vi "Get Joystick Output.vi"(0 "JoystickDevRef":T1={"Device"=enum."USB 1"}, 11 "error in (no error)":errorcluster) -> (3 "XBox?":bool, 4 "JoystickDevRef":T1, 6 "Axes":dbl[](array[numeric]), 8 "Buttons":bool[](array[boolean]), 10 "POVs":i16[](array[numeric]), 15 "error out":errorcluster)   [LabVIEW 2014]
uses:
  <vilib>/Rock Robotics/WPI/Joystick/WPI_JoystickDevRef.ctl
  <vilib>/Rock Robotics/WPI/Joystick/WPI_JoystickDeviceEnum.ctl
  <vilib>/Rock Robotics/WPI/Joystick/WPI_JoystickXBox Types.ctl
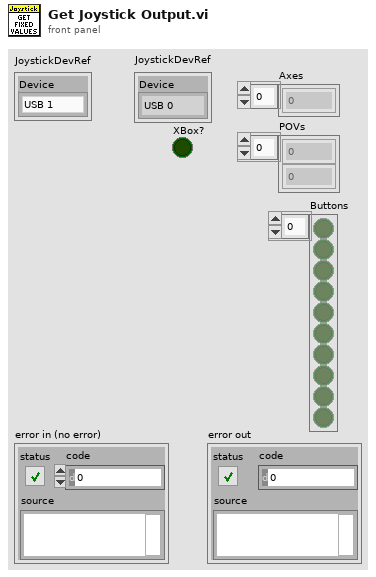
[diagram p1: front panel]
types:
  T1 = typedef "WPI_JoystickDevRef.ctl" = cluster{"Device":T2}
  T2 = typedef "WPI_JoystickDeviceEnum.ctl" = enum16{"USB 0", "USB 1", "USB 2", "USB 3", "USB 4", "USB 5"}
  T3 = typedef "WPI_JoystickXBox Types.ctl" = enum16{"Not XBox", "XBox Unknown", "XBox Gamepad", "XBox Wheel", "XBox Arcade Stick", "XBox Flight Stick", "XBox Dance Pad", "XBox Guitar", "XBox Drum Kit", "XBox Arcade Pad"}
  T4 = typedef "WPI_Joystick Info.ctl" = cluster{"Device Name":string, "HID Type":T5, "XBox Type":T3, "Axes Count":i32, "Axes Types":T6[], "Button Count":i32, "POV Count":i32}
  T5 = typedef "WPI_JoystickHID Types.ctl" = enum16{"Not HID", "HID Joystick", "HID Gamepad", "HID Driving Wheel", "HID Flightstick", "HID First Person"}
  T6 = typedef "WPI_JoystickAxis Types.ctl" = enum16{"X Axis", "Y Axis", "Z Axis", "RxAxis", "RyAxis", "RzAxis", "Slider", "POV", "None", "L X Axis", "L Y Axis", "L Trigger", "R Trigger", "R X Axis", "R Y Axis"}
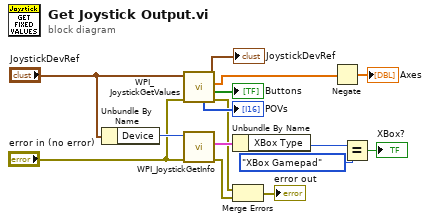
[diagram p0: block diagram]
diagram:
  n1 = Unbundle By Name("JoystickDevRef") -> ("Device"=w14:T2)
  n2 = call <vilib>:"WPI_JoystickGetValues.vi"("error in (no error)"="error in (no error)", "JoystickDevRef"="JoystickDevRef") -> ("error out"=w9:errorcluster, "Buttons"=→"Buttons":bool[], "Axes"=w5:dbl[], "JoystickDevRef"=→"JoystickDevRef":T1, "POVs"=→"POVs":i16[])  [unwired: 5 in]
  n3 = call <vilib>:"WPI_JoystickGetInfo.vi"("error in (no error)"="error in (no error)", "JoystickDevice"=w14) -> ("error out"=w8:errorcluster, "Joystick Info"=w13:T4)  [unwired: 8 in]
  n4 = Unbundle By Name(w13) -> ("XBox Type"=w3:T3)
  n5 = Merge Errors(w9, w8) -> (→"error out":errorcluster)
  n6 = Negate(x=w5) -> (-x=→"Axes":dbl[])
  n7 = Equal?(x=w3, y=WPI_JoystickXBox_Types."XBox Gamepad") -> (x = y?=→"XBox?":bool)
